vi "S2C_SaveSubScript.vi"(8 "Error In":errorcluster) -> (0 "Error Out":errorcluster, 3 "Cancel?":bool)   [LabVIEW 2015]
doc: "Deletes the selected items from the script table."
uses:
  Globals/S2C_Globals.vi
  <vilib>/Utility/config.llb/Write Key (String).vi
  <vilib>/Utility/config.llb/NI_LVConfig.lvlib
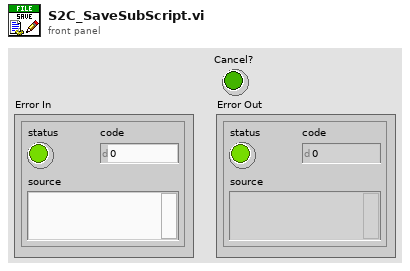
[diagram p1: front panel]
types:
  T1 = typedef "NI_LVConfig.lvlib/Config Data RefNum.ctl" = refnum<k1>
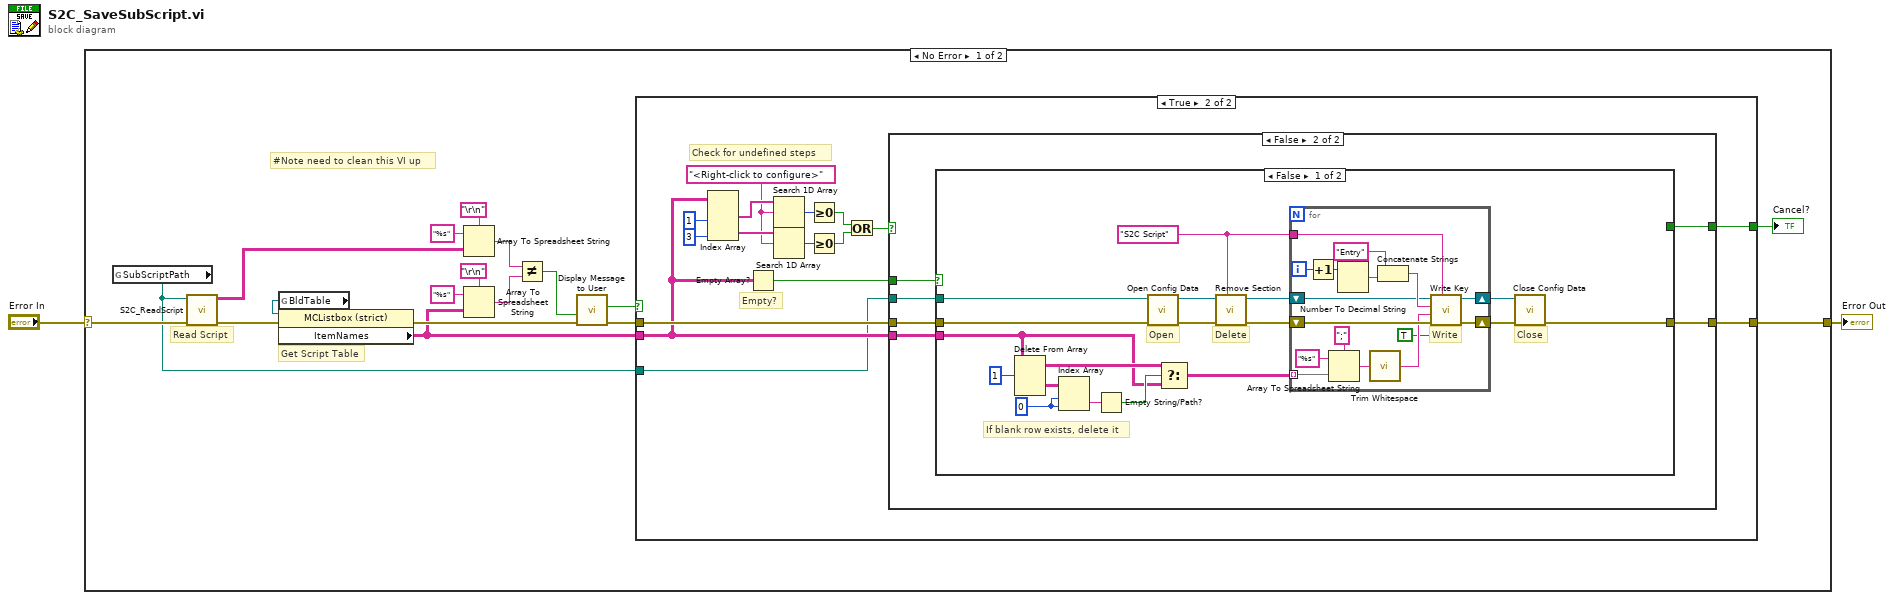
[diagram p0: block diagram]
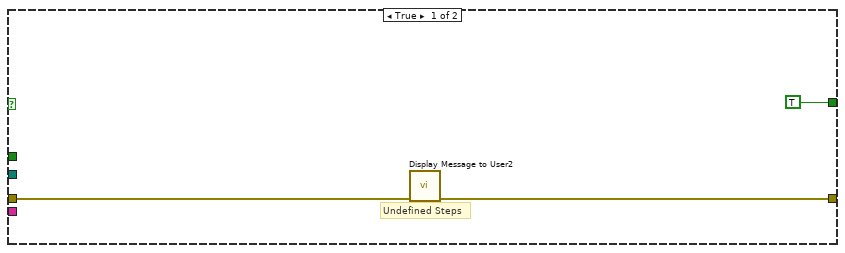
[diagram p3: hidden frame]
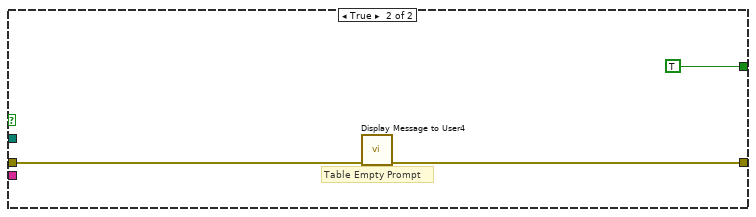
[diagram p4: hidden frame]
diagram:
  n1 = case shown="No Error" "Error In" {
    selector: "Error In" -> [w14 w84]
    tunnel: [w4 w84] -> w1
    frame No Error {
      # "#Note need to clean this VI up"
      # "Read Script"
      # "Get Script Table"
      n2 = global read "S2C_Globals.vi" "SubScriptPath"() -> (w5:path)
      n3 = call "S2C_ReadScript.vi"("Error In"=w14, "FilePath"=w5) -> ("Error Out"=w13:errorcluster, "Data"=w10:string[][])  [unwired: 8 in]
      n4 = global read "S2C_Globals.vi" "BldTable"() -> (w20:refnum<vi>)
      n5 = property class="MCListbox (strict)"(reference=w20, error in=w13) -> (error out=w16:errorcluster, "ItemNames"=w6:string[][])  [unwired: 1 out]
      n6 = Array To Spreadsheet String(delimiter (Tab)="\r\n", array=w10, 3:"%s" ("format string")) -> (spreadsheet string=w9:string)
      n7 = Array To Spreadsheet String(delimiter (Tab)="\r\n", array=w6, 3:"%s" ("format string")) -> (spreadsheet string=w17:string)
      n8 = Not Equal?(x=w9, y=w17) -> (x != y?=w15:bool)
      n9 = call "Display Message to User"("error in (no error)"=w16, "Enable"=w15) -> ("error out"=w8:errorcluster, "Yes"=w7:bool)  [unwired: 8 in]
      n10 = case shown="True" w7 {
        tunnel: w8 -> [w21 w34]
        tunnel: w6 -> [_ w33]
        tunnel: w5 -> [_ w32]
        tunnel: [w21 w23] -> w4
        tunnel: [_ w22] -> w3
        frame False {
          # "No Changes Saved"
        }
        frame True {
          w24 = "<Right-click to configure>"
          # "Check for undefined steps"
          # "Empty?"
          n11 = Index Array(array=w33, index (col) #1=1 ("disabled index (col)"), index (col) #2=3 ("index (col)")) -> (element #1=w36:string[], element #2=w30:string[])  [unwired: 2 in]
          n12 = Empty Array?(array=w33) -> (empty?=w35:bool)
          n13 = Search 1D Array(1D array=w36, element=w24) -> (index of element=w29:i32)  [unwired: 1 in]
          n14 = Search 1D Array(1D array=w30, element=w24) -> (index of element=w28:i32)  [unwired: 1 in]
          n15 = Greater Or Equal To 0?(x=w29) -> (x >= 0?=w27:bool)
          n16 = Greater Or Equal To 0?(x=w28) -> (x >= 0?=w26:bool)
          n17 = Or(x=w27, y=w26) -> (x .or. y?=w25:bool)
          n18 = case shown="False" w25 {
            tunnel: w34 -> [w39 w46]
            tunnel: [w40 w45] -> w23
            tunnel: w32 -> [_ w43]
            tunnel: w33 -> [_ w44]
            tunnel: w35 -> [_ w42]
            tunnel: [TRUE w41] -> w22
            frame True {
              # "Undefined Steps"
              n19 = call "Display Message to User2"("error in (no error)"=w39) -> ("error out"=w40:errorcluster)  [unwired: 9 in, 1 out]
            }
            frame False {
              n20 = case shown="False" w42 {
                tunnel: w46 -> [w61 w83]
                tunnel: [w47 w82] -> w45
                tunnel: w44 -> [w49 _]
                tunnel: w43 -> [w48 _]
                tunnel: [_ TRUE] -> w41
                frame False {
                  w56 = 0 ("index (row)")
                  w50 = "S2C Script"
                  # "If blank row exists, delete it"
                  # "Delete"
                  # "Close"
                  # "Open"
                  n21 = Delete From Array(array=w49, length=1) -> (deleted portion=w57:string[][], array with subset deleted=w59:string[][])  [unwired: 2 in]
                  n22 = Index Array(array=w57, index (row)=w56, index (col)=w56) -> (element=w55:string)
                  n23 = Empty String/Path?(string/path=w55) -> (empty?=w54:bool)
                  n24 = call <vilib>:"Open Config Data.vi"("error in (no error)"=w61, "configuration file path"=w48) -> ("error out"=w64:errorcluster, "refnum"=w52:T1)  [unwired: 7 in, 1 out]
                  n25 = Select(t=w59, s=w54, f=w49) -> (s? t:f=w58:string[][])
                  n26 = call <vilib>:"Remove Section.vi"("section"=w50, "error in (no error)"=w64, "refnum"=w52) -> ("error out"=w53:errorcluster, "refnum out"=w51:T1)  [unwired: 6 in, 1 out]
                  n27 = for {
                    tunnel: w58 -> [w80] mode=indexing
                    shift-right: [w72] -> w63
                    shift-left: w53 -> [w73]
                    tunnel: w50 -> [w69]
                    shift-right: [w67] -> w62
                    shift-left: w51 -> [w68]
                    i -> [w78]
                    # "Write"
                    n28 = Increment(x=w78) -> (x+1=w77:i32)
                    n29 = Array To Spreadsheet String(delimiter (Tab)=";", array=w80, 3:"%s" ("format string")) -> (spreadsheet string=w71:string)
                    n30 = Number To Decimal String(number=w77) -> (decimal integer string=w75:string)  [unwired: 1 in]
                    n31 = call <vilib>:"Trim Whitespace.vi"("string"=w71) -> ("trimmed string"=w66:string)  [unwired: 1 in]
                    n32 = Concatenate Strings("Entry" ("string"), w75) -> (w70:string)
                    n33 = call-poly <vilib>:"Write Key.vi"("write raw string? (F)"=TRUE, "section"=w69, "error in (no error)"=w73, "value"=w66, "key"=w70, "refnum"=w68) -> ("error out"=w72:errorcluster, "refnum out"=w67:T1)  [unwired: 3 in, 1 out]
                  }
                  n34 = call <vilib>:"Close Config Data.vi"("error in (no error)"=w63, "refnum"=w62) -> ("error out"=w47:errorcluster)  [unwired: 8 in, 1 out]
                }
                frame True {
                  # "Table Empty Prompt"
                  n35 = call "Display Message to User4"("error in (no error)"=w83) -> ("error out"=w82:errorcluster)  [unwired: 9 in, 1 out]
                }
              }
            }
          }
        }
      }
      "Cancel?" <- w3
    }
    frame Error {
    }
  }
  "Error Out" <- w1
